vi "Write Work FIFO.vi"(8 "error in (no error)":errorcluster, 9 "timeout in ms (0)":i32 format="%d ms", 10 "command in":T1, 11 "Work FIFO in":refnum<k33>) -> (0 "error out":errorcluster, 1 "timed out?":bool, 2 "command out":T1, 3 "Work FIFO out":refnum<k33>, 4 "# elements":u32)   [LabVIEW 2017, in "DSF Core.lvlib" / "Dispatcher.lvclass"]
uses:
  Dispatcher.lvclass
  Interfaces/Dispatcher/Command Data.ctl
  Interfaces/Dispatcher/Command.ctl
  Interfaces/Dispatcher/Parameters.ctl
  Interfaces/Dispatcher/Dispatcher Interface.lvclass
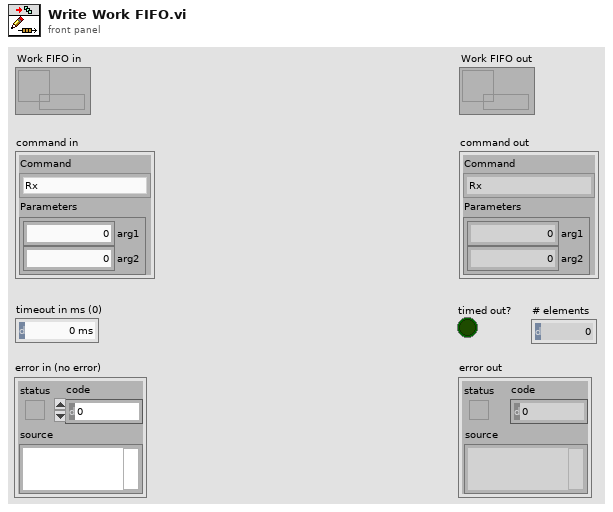
[diagram p1: front panel]
types:
  T1 = typedef "DSF Core.lvlib/Dispatcher Interface.lvclass/Command Data.ctl" = cluster{"Command":T2, "Parameters":T3}
  T2 = typedef "DSF Core.lvlib/Dispatcher Interface.lvclass/Command.ctl" = enum8{"Rx", "Tx", "Shutdown"}
  T3 = typedef "DSF Core.lvlib/Dispatcher Interface.lvclass/Parameters.ctl" = cluster{"arg1":u64, "arg2":u64}
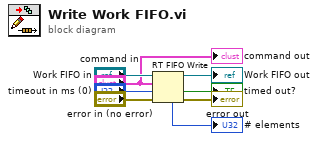
[diagram p0: block diagram]
diagram:
  n1 = RT FIFO Write(0:"Work FIFO in", 1:"command in", 2:"timeout in ms (0)", 3:"error in (no error)") -> (7:→"# elements":u32, 8:→"Work FIFO out":refnum<k33>, 10:→"timed out?":bool, 11:→"error out":errorcluster)  [unwired: 1 in]
  "command out" <- "command in"
